vi "Read Unique ID.vi"(11 "Topic in":refnum<class "Topic.lvclass">) -> (3 "Unique ID":string)   [LabVIEW 2015, in "Mediator.lvlib" / "Topic.lvclass"]
uses:
  Topic.lvclass
  <vilib>/ActorFramework/Actor/Actor.lvclass/Actor.ctl
  <vilib>/ActorFramework/Message Enqueuer/Message Enqueuer.lvclass/Message Enqueuer.ctl
  <vilib>/ActorFramework/Message Enqueuer/Init from Existing Queue.vi
  <vilib>/ActorFramework/Message Enqueuer/Message Enqueuer.lvclass
  <vilib>/ActorFramework/Actor/Actor.lvclass
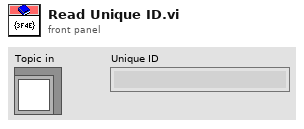
[diagram p1: front panel]
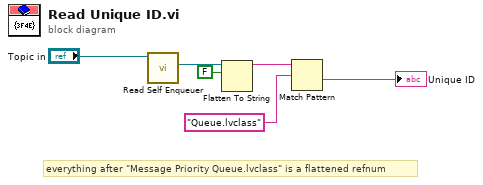
[diagram p0: block diagram]
diagram:
  # "everything after \"Message Priority Queue.lvclass\" is a flattened refnum"
  n1 = call <vilib>:"Read Self Enqueuer.vi"("Actor"="Topic in") -> ("Self Enqueuer"=w6:refnum<class "Message Enqueuer.lvclass">)  [unwired: 10 in]
  n2 = Flatten To String(anything=w6, prepend array or string size? (T)=FALSE) -> (data string=w5:string)  [unwired: 2 in, 2 out]
  n3 = Match Pattern(string=w5, regular expression="Queue.lvclass") -> (after substring=→"Unique ID":string)  [unwired: 1 in, 3 out]
